vi "lab #5 (while loop with signal).vi"() -> ()   [LabVIEW 2016]
panel:
  in  "x":bool
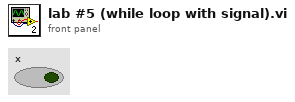
[diagram p1: front panel]
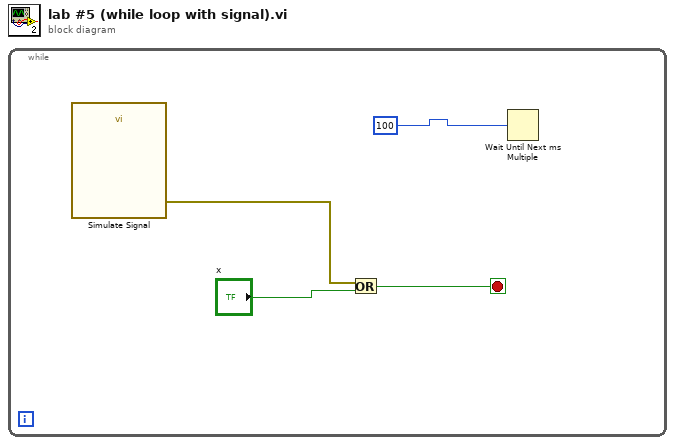
[diagram p0: block diagram]
diagram:
  n1 = while {
    stop <- w4 stop-if-true
    n2 = call "Simulate Signal"() -> ("error out"=w2:errorcluster)  [unwired: 14 in, 1 out]
    n3 = Or(x=w2, y="x") -> (x .or. y?=w4:bool)
    n4 = Wait Until Next ms Multiple(millisecond multiple=u32 100 ("millisecond timer value")) -> ()  [unwired: 1 out]
  }
